vi "State_Machine.vi"   [LabVIEW 2018]
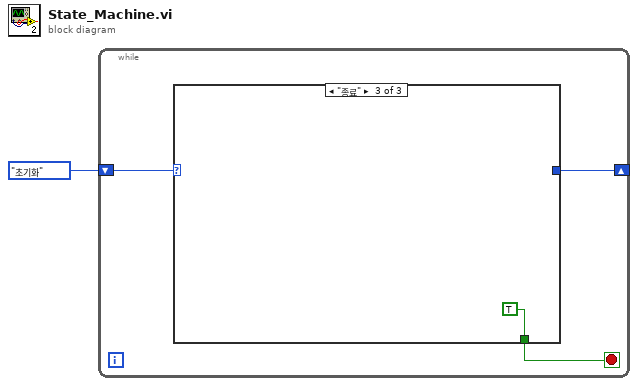
[diagram p0: block diagram]
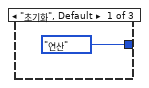
[diagram p2: hidden frame]
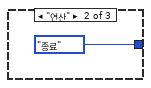
[diagram p3: hidden frame]
diagram:
  n1 = while {
    shift-right: [w3] -> _
    shift-left: enum16{"초기화", "연산", "종료"}."초기화" -> [w4]
    stop <- w2 stop-if-true
    n2 = case shown="\"종료\"" w4 {
      tunnel: [enum16{"초기화", "연산", "종료"}."연산" enum16{"초기화", "연산", "종료"}."종료" _] -> w3
      tunnel: [_ _ TRUE] -> w2
      frame "초기화", Default {
      }
      frame "연산" {
      }
      frame "종료" {
      }
    }
  }
